vi "Close.vi"(8 "error in (no error)":errorcluster, 11 "InfoService in":refnum<class "NodeStatus.lvclass">) -> (0 "error out":errorcluster)   [LabVIEW 2020, in "Vecto.lvlib" / "NodeStatus.lvclass"]
uses:
  NodeStatus.lvclass
  NodeStatus.lvclass/NodeStatus.ctl
panel:
  out "call chain":string[](array[string])
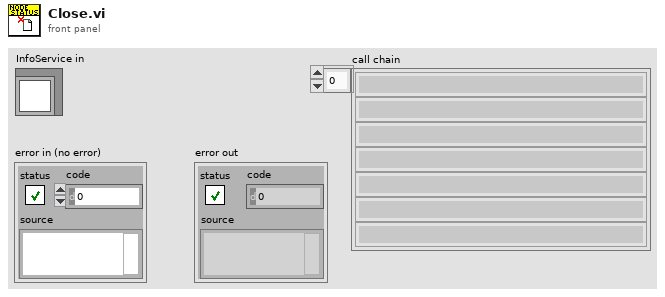
[diagram p1: front panel]
types:
  T1 = typedef "Vecto.lvlib/NodeStatus.lvclass/Incoming Events.ctl" = cluster{"Info Request":refnum<user-event>, "Update Task":refnum<user-event>, "Update Info":refnum<user-event>, "Close":refnum<user-event>}
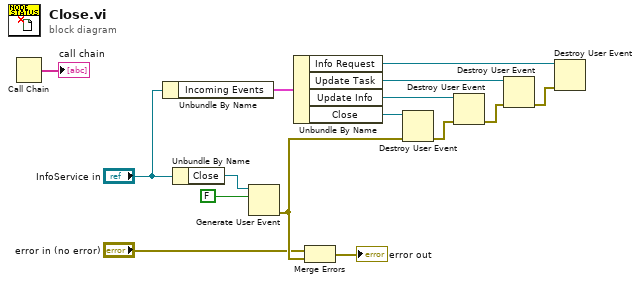
[diagram p0: block diagram]
diagram:
  n1 = Call Chain() -> (call chain=→"call chain":string[])
  n2 = Unbundle By Name("InfoService in") -> ("Incoming Events"=w12:T1)
  n3 = Unbundle By Name("InfoService in") -> ("Close"=w15:refnum<user-event>)
  n4 = Generate User Event(user event=w15, event data cluster=FALSE ("event data")) -> (error out=w10:errorcluster)  [unwired: 2 in, 1 out]
  n5 = Unbundle By Name(w12) -> ("Info Request"=w2:refnum<user-event>, "Update Task"=w4:refnum<user-event>, "Update Info"=w7:refnum<user-event>, "Close"=w11:refnum<user-event>)
  n6 = Merge Errors("error in (no error)", w10) -> (→"error out":errorcluster)
  n7 = Destroy User Event(user event=w11, error in=w10) -> (error out=w6:errorcluster)
  n8 = Destroy User Event(user event=w7, error in=w6) -> (error out=w3:errorcluster)
  n9 = Destroy User Event(user event=w4, error in=w3) -> (error out=w5:errorcluster)
  n10 = Destroy User Event(user event=w2, error in=w5) -> ()  [unwired: 1 out]
